vi "Example RX.vi"(0 "niInstr Network API FPGA v1.lvclass":refnum<class "niInstr Network API FPGA v1.lvclass">, 1 "Port RX Clear Counts":bool, 2 "Host RX FIFO":refnum<k21>, 7 "RAW Mode":bool, 11 "Dest Port":u16) -> (4 "debug data":T1)   [LabVIEW 2020, in "My Network FPGA v1.lvlib"]
uses:
  My Network FPGA v1.lvlib
  <instrlib>/_niInstr/Network/API/v1/FPGA/niInstr Network API FPGA v1.lvclass
  <instrlib>/_niInstr/Network/Ethernet/MAC/Data Stream/v1/Read Data Stream.vi
  <instrlib>/_niInstr/Network/Ethernet/MAC/Data Stream/v1/Read End of Good Frame.vi
  <instrlib>/_niInstr/Basic Elements/v1/FPGA/Private/Count Up U32.vi
  <instrlib>/_niInstr/Network/Ethernet/MAC/Data Stream/v1/Read End of Bad Frame.vi
  <instrlib>/_niInstr/Network/IPv4/UDP/Data Stream/v1/Read Data Stream.vi
  <vilib>/rvi/DataTransferAndStorage/Container/Common/niFpgaContainerExecOnDevCompGetState.vi
  <vilib>/rvi/Emulation/niFpgaSctlEmulationGetInTimedLoop.vi
  <vilib>/rvi/errors/niFpgaSetErrorForExecOnDevCompSimple.vi
  <vilib>/rvi/eio/common/nirviEmuReportErrorAndStop.vi
  <vilib>/rvi/interface/RandomDataEmulation/nirviRandomDataAcquireLock.vi
  <vilib>/rvi/interface/RandomDataEmulation/nirviRandomDataQueueStore.vi
  <vilib>/rvi/interface/RandomDataEmulation/nirviRandomDataReleaseLock.vi
  <vilib>/rvi/interface/RandomDataEmulation/nirviFPGAContextMergeError.vi
  <vilib>/rvi/interface/RandomDataEmulation/nirviRandomDataCheckExitLoopConditions.vi
  <vilib>/express/rvi/timingcommon/nirviCommon.vi
  <vilib>/rvi/interface/RandomDataEmulation/niFpgaRandomDataHandleErrors.vi
  <vilib>/rvi/DataTransferAndStorage/Container/XNode/niFpgaContainer.xnode
  <vilib>/rvi/FIFO/Fifo_Resource/niFpgaFifoEmulationRefInMultiElement.vi
  <instrlib>/_niInstr/Network/Ethernet/MAC/Data Stream/v1/niInstr Ethernet MAC Data Stream v1.lvclass
  <instrlib>/_niInstr/Network/IPv4/UDP/Data Stream/v1/niInstr IPv4 UDP Data Stream v1.lvclass
  <instrlib>/_niInstr/Basic Elements/v1/FPGA/niInstr Basic Elements v1 FPGA.lvlib
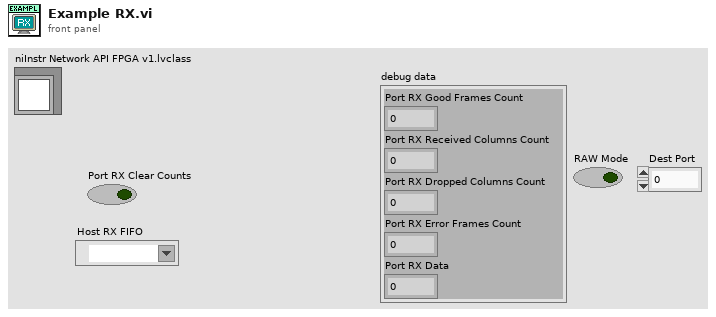
[diagram p1: front panel]
types:
  T1 = cluster{"Port RX Good Frames Count":u32, "Port RX Received Columns Count":u32, "Port RX Dropped Columns Count":u32, "Port RX Error Frames Count":u32, "Port RX Data":u64}
  T2 = typedef "niInstr Ethernet Utilities FPGA v1.lvlib/Network Data Stream.ctl" = cluster{"data":u8[], "data valid":bool, "byte enables":bool[]}
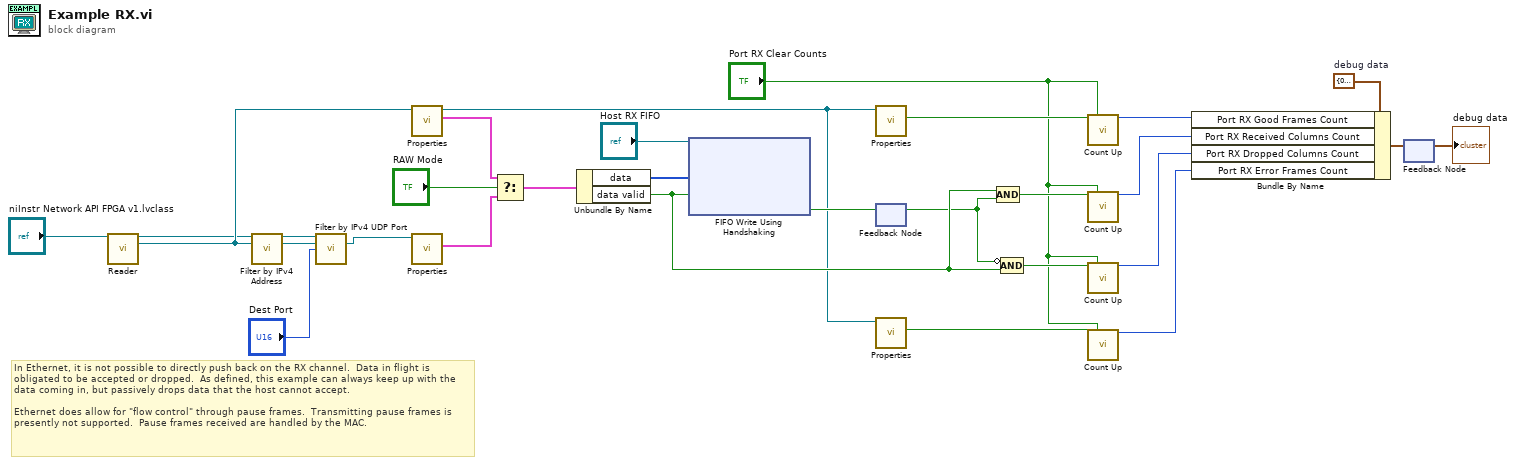
[diagram p0: block diagram]
diagram:
  w28 = T1 {"Port RX Good Frames Count"=0, "Port RX Received Columns Count"=0, "Port RX Dropped Columns Count"=0, "Port RX Error Frames Count"=0, "Port RX Data"=0}  # debug data
  # "In Ethernet, it is not possible to directly push back on the RX channel.  Data in flight is obligated to be accepted or dropped.  As defined, this example can always keep up with the data coming in, but passively drops data that the host cannot accept.\n\nEthernet does allow for \"flow control\" through pause frames.  Transmitting pause frames is presently not supported.  Pause frames received are handled by the MAC."
  n1 = call <instrlib>:"Reader.vi"("niInstr Network API FPGA v1.lvclass"="niInstr Network API FPGA v1.lvclass") -> ("niInstr Network API FPGA v1.lvclass out"=w6:refnum<class "niInstr Network API FPGA v1.lvclass">, "niInstr Ethernet MAC Data Stream v1 out"=w7:refnum<class "niInstr Ethernet MAC Data Stream v1.lvclass">)  [unwired: 13 in]
  n2 = call <instrlib>:"Filter by IPv4 Address.vi"("niInstr Network API FPGA v1 in"=w6, "niInstr Ethernet MAC Data Stream v1 in"=w7) -> ("niInstr Network API FPGA v1 out"=w5:refnum<class "niInstr Network API FPGA v1.lvclass">, "niInstr IPv4 Data Stream out"=w4:refnum<class "niInstr IPv4 Data Stream v1.lvclass">)  [unwired: 12 in]
  n3 = call <instrlib>:"Filter by IPv4 UDP Port.vi"("niInstr Network API FPGA v1 in"=w5, "niInstr IPv4 Data Stream in"=w4, "Dest Port"="Dest Port") -> ("niInstr IPv4 UDP Data Stream out"=w3:refnum<class "niInstr IPv4 UDP Data Stream v1.lvclass">)  [unwired: 11 in, 1 out]
  n4 = call-poly <instrlib>:"Properties.vi"("niInstr Ethernet MAC Data Stream v1 in"=w7) -> ("Data Stream"=w21:T2, "niInstr Ethernet MAC Data Stream v1 out"=w9:refnum<class "niInstr Ethernet MAC Data Stream v1.lvclass">)  [unwired: 9 in]
  n5 = call-poly <instrlib>:"Properties.vi"("niInstr IPv4 UDP Data Stream v1.lvclass"=w3) -> ("Data Stream"=w19:T2)  [unwired: 9 in, 1 out]
  n6 = Select(t=w21, s="RAW Mode", f=w19) -> (s? t:f=w20:T2)
  n7 = Unbundle By Name(w20) -> ("data"=w25:u8[], "data valid"=w24:bool)
  n8 = xnode ("FIFO Write Using Handshaking")("Element"=w25, "Input Valid"=w24, "FIFO In"="Host RX FIFO") -> ("Ready for Input"=w23:bool)  [unwired: 1 out]
  n9 = call-poly <instrlib>:"Properties.vi"("niInstr Ethernet MAC Data Stream v1 in"=w9) -> ("End of Good Frame"=w18:bool)  [unwired: 9 in, 1 out]
  n10 = feedback #1() -> (w22:bool)  [unwired: 1 in]
  n11 = feedback-in #1(w23) -> ()
  n12 = call-poly <instrlib>:"Properties.vi"("niInstr Ethernet MAC Data Stream v1 in"=w9) -> ("End of Bad Frame"=w12:bool)  [unwired: 9 in, 1 out]
  n13 = Compound Arithmetic op=AND(w24, w22) -> (w16:bool)
  n14 = Compound Arithmetic op=AND(invert w22, w24) -> (w14:bool)
  n15 = call-poly <instrlib>:"Count Up.vi"("increment"=w18, "reset"="Port RX Clear Counts") -> ("count out"=w17:u32)  [unwired: 13 in]
  n16 = call-poly <instrlib>:"Count Up.vi"("increment"=w16, "reset"="Port RX Clear Counts") -> ("count out"=w15:u32)  [unwired: 13 in]
  n17 = call-poly <instrlib>:"Count Up.vi"("increment"=w14, "reset"="Port RX Clear Counts") -> ("count out"=w13:u32)  [unwired: 13 in]
  n18 = call-poly <instrlib>:"Count Up.vi"("increment"=w12, "reset"="Port RX Clear Counts") -> ("count out"=w11:u32)  [unwired: 13 in]
  n19 = Bundle By Name(cluster=w28, "Port RX Good Frames Count"=w17, "Port RX Received Columns Count"=w15, "Port RX Dropped Columns Count"=w13, "Port RX Error Frames Count"=w11) -> (w29:T1)
  n20 = feedback-in #2(w29) -> ()
  n21 = feedback #2() -> (→"debug data":T1)  [unwired: 1 in]
